vi "Pratik3-Case2 (SubVI).vi"(1 "Dalga Fazı(’C)":dbl min=0.0 max=360.0 step=1.0, 2 "Dalga Frekansı(Hz)":dbl=40.0 min=40.0 step=1000000.0 format="%#_9g", 3 "Dalga Genliği(mV)":dbl min=0.0 max=376000.0 step=11.5, 4 "Dalga Şekli":enum16{"Kare", "Üçgen", "Sinüs", "Testere Dişi"}(ring)) -> (0 "MESSAGE":string)   [LabVIEW 2024]
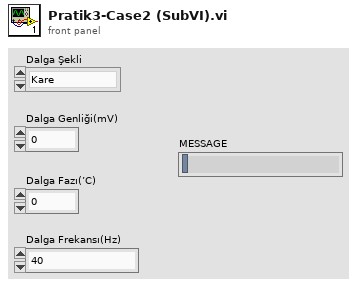
[diagram p1: front panel]
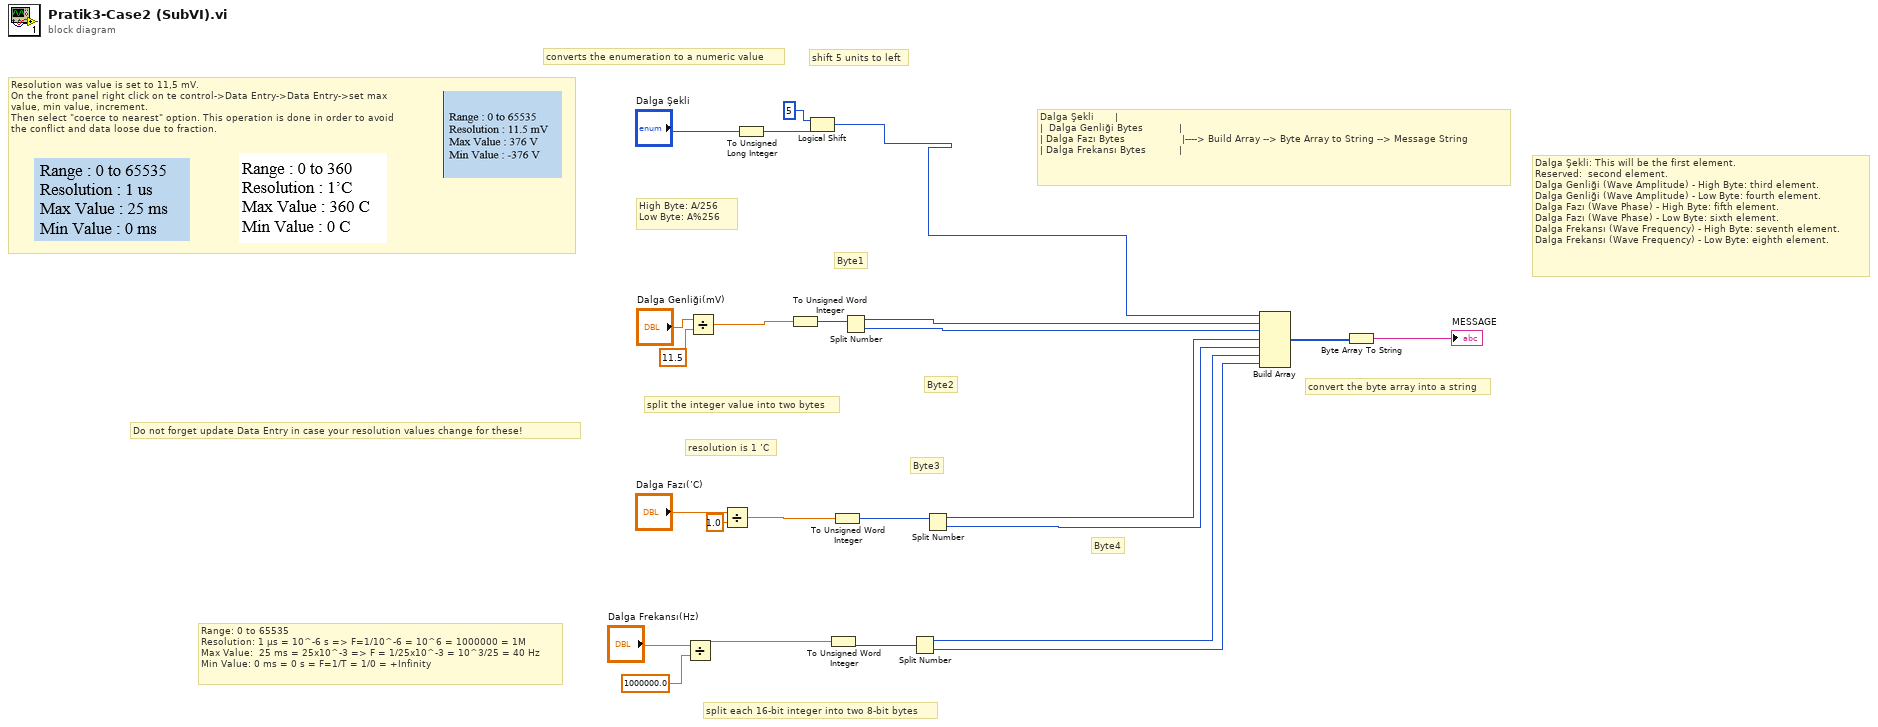
[diagram p0: block diagram]
diagram:
  # "Do not forget update Data Entry in case your resolution values change for these!"
  # "Range: 0 to 65535\nResolution: 1 µs = 10^-6 s => F=1/10^-6 = 10^6 = 1000000 = 1M\nMax Value:  25 ms = 25x10^-3 => F = 1/25x10^-3 = 10^3/25 = 40 Hz\nMin Value: 0 ms = 0 s = F=1/T = 1/0 = +Infinity"
  # "resolution is 1 ’C"
  # "Resolution was value is set to 11,5 mV.\nOn the front panel right click on te control->Data Entry->Data Entry->set max \nvalue, min value, increment.\nThen select \"coerce to nearest\" option. This operation is done in order to avoid \nthe conflict and data loose due to fraction."
  # "High Byte: A/256\nLow Byte: A%256"
  # "Dalga Şekli: This will be the first element.\nReserved:  second element.\nDalga Genliği (Wave Amplitude) - High Byte: third element.\nDalga Genliği (Wave Amplitude) - Low Byte: fourth element.\nDalga Fazı (Wave Phase) - High Byte: fifth element.\nDalga Fazı (Wave Phase) - Low Byte: sixth element.\nDalga Frekansı (Wave Frequency) - High Byte: seventh element.\nDalga Frekansı (Wave Frequency) - Low Byte: eighth element."
  # "Dalga Şekli       |\n|  Dalga Genliği Bytes            |        \n| Dalga Fazı Bytes                   |----> Build Array --> Byte Array to String --> Message String\n| Dalga Frekansı Bytes           |"
  # "convert the byte array into a string"
  # "split each 16-bit integer into two 8-bit bytes"
  # "split the integer value into two bytes"
  # "Byte4"
  # "Byte3"
  # "Byte2"
  # "Byte1"
  # "shift 5 units to left"
  # "converts the enumeration to a numeric value"
  n1 = Divide(x="Dalga Frekansı(Hz)", y=1000000.0) -> (x/y=w24:dbl)
  n2 = Divide(x="Dalga Genliği(mV)", y=11.5) -> (x/y=w16:dbl)
  n3 = Divide(x="Dalga Fazı(’C)", y=1.0) -> (x/y=w4:dbl)
  n4 = To Unsigned Long Integer(number="Dalga Şekli") -> (unsigned 32bit integer=w8:u32)
  n5 = To Unsigned Word Integer(number=w16) -> (unsigned 16bit integer=w17:u16)
  n6 = Logical Shift(y=i16 5, x=w8) -> (x << y=w21:u32)
  n7 = To Unsigned Word Integer(number=w24) -> (unsigned 16bit integer=w6:u16)
  n8 = To Unsigned Word Integer(number=w4) -> (unsigned 16bit integer=w5:u16)
  n9 = Split Number(x=w17) -> (hi(x)=w18:u8, lo(x)=w19:u8)
  n10 = Split Number(x=w6) -> (hi(x)=w10:u8, lo(x)=w11:u8)
  n11 = Split Number(x=w5) -> (hi(x)=w12:u8, lo(x)=w9:u8)
  n12 = Build Array "Build Array"(w21, w18, w19, w12, w9, w10, w11) -> (w13:u32[])
  n13 = Byte Array To String(unsigned byte array=w13) -> (string=→"MESSAGE":string)
